vi "Calculate_dx_dy_alpha.vi"(6 "c_y":dbl, 7 "c_x":dbl, 8 "Corresponding Point #2":i32, 9 "Corresponding Point #1":i32, 10 "Original Plots":T1(array[cluster]), 11 "Captured Plots":T1(array[cluster])) -> (1 "alpha":dbl, 2 "dy":dbl, 3 "dx":dbl)   [LabVIEW 2012]
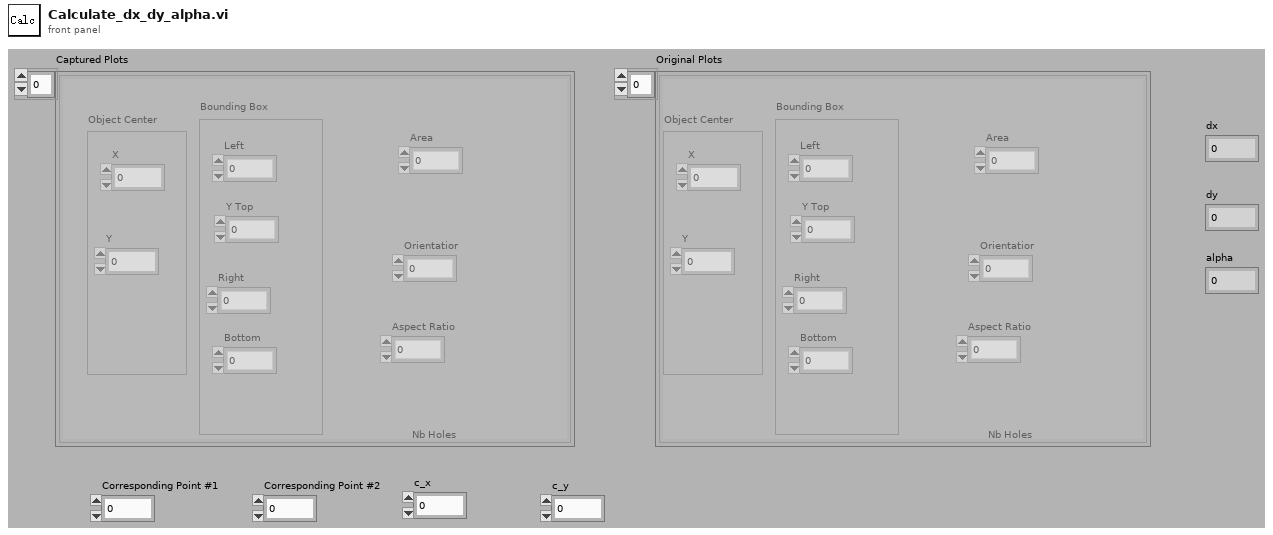
[diagram p1: front panel]
types:
  T1 = cluster{"Object Center":cluster{"X":dbl, "Y":dbl}, "Bounding Box":cluster{"Left":dbl, "Right":dbl, "Bottom":dbl, "Y Top":dbl}, "Area":dbl, "Orientatior":dbl, "Aspect Ratio":dbl, "Nb Holes":dbl}[]
  T2 = cluster{"Object Center":cluster{"X":dbl, "Y":dbl}, "Bounding Box":cluster{"Left":dbl, "Right":dbl, "Bottom":dbl, "Y Top":dbl}, "Area":dbl, "Orientatior":dbl, "Aspect Ratio":dbl, "Nb Holes":dbl}
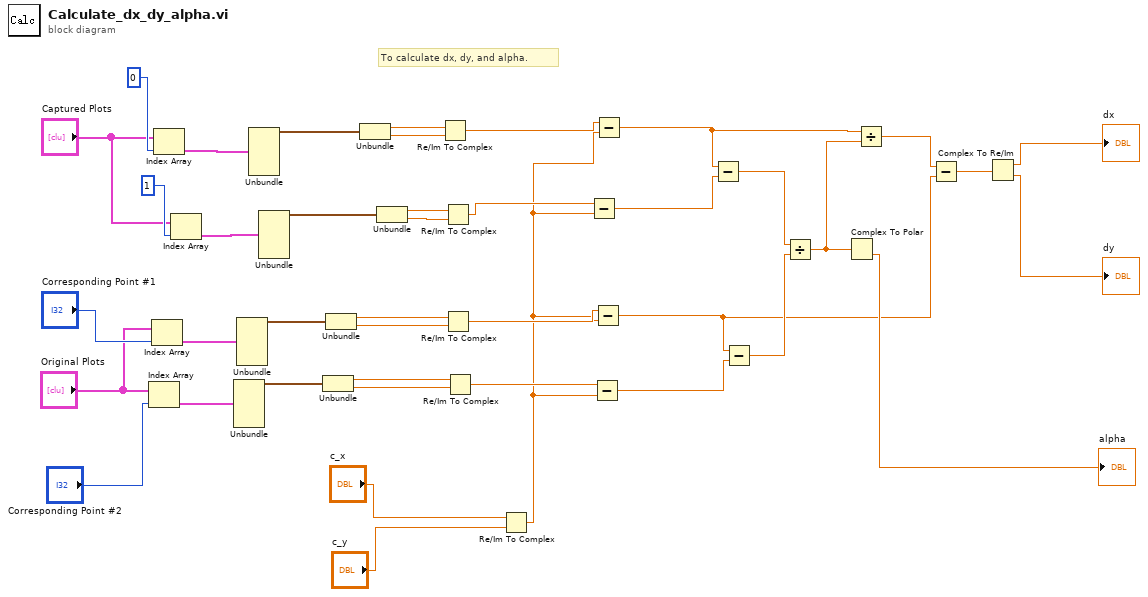
[diagram p0: block diagram]
diagram:
  # "To calculate dx, dy, and alpha."
  n1 = Index Array(array="Original Plots", index="Corresponding Point #2") -> (element=w37:T2)
  n2 = Index Array(array="Original Plots", index="Corresponding Point #1") -> (element=w35:T2)
  n3 = Index Array(array="Captured Plots", index=0) -> (element=w40:T2)
  n4 = Index Array(array="Captured Plots", index=1) -> (element=w31:T2)
  n5 = Unbundle(w37) -> ("Object Center"=w38:cluster{"X":dbl, "Y":dbl})  [unwired: 5 out]
  n6 = Unbundle(w35) -> ("Object Center"=w36:cluster{"X":dbl, "Y":dbl})  [unwired: 5 out]
  n7 = Unbundle(w40) -> ("Object Center"=w39:cluster{"X":dbl, "Y":dbl})  [unwired: 5 out]
  n8 = Unbundle(w31) -> ("Object Center"=w30:cluster{"X":dbl, "Y":dbl})  [unwired: 5 out]
  n9 = Unbundle(w38) -> ("X"=w19:dbl, "Y"=w18:dbl)
  n10 = Unbundle(w36) -> ("X"=w21:dbl, "Y"=w20:dbl)
  n11 = Unbundle(w39) -> ("X"=w25:dbl, "Y"=w24:dbl)
  n12 = Unbundle(w30) -> ("X"=w23:dbl, "Y"=w22:dbl)
  n13 = Re/Im To Complex(1:w24, 2:w25) -> (0:w17:cdb)
  n14 = Re/Im To Complex(1:w22, 2:w23) -> (0:w16:cdb)
  n15 = Re/Im To Complex(1:w20, 2:w21) -> (0:w15:cdb)
  n16 = Re/Im To Complex(1:w18, 2:w19) -> (0:w14:cdb)
  n17 = Re/Im To Complex(1:"c_y", 2:"c_x") -> (0:w13:cdb)
  n18 = Subtract(x=w16, y=w13) -> (x-y=w12:cdb)
  n19 = Subtract(x=w14, y=w13) -> (x-y=w11:cdb)
  n20 = Subtract(x=w15, y=w13) -> (x-y=w4:cdb)
  n21 = Subtract(x=w17, y=w13) -> (x-y=w7:cdb)
  n22 = Subtract(x=w7, y=w12) -> (x-y=w10:cdb)
  n23 = Subtract(x=w4, y=w11) -> (x-y=w9:cdb)
  n24 = Divide(x=w10, y=w9) -> (x/y=w6:cdb)
  n25 = Complex To Polar(r * e^(i*theta)=w6) -> (theta=→"alpha":dbl)  [unwired: 1 out]
  n26 = Divide(x=w7, y=w6) -> (x/y=w5:cdb)
  n27 = Subtract(x=w5, y=w4) -> (x-y=w3:cdb)
  n28 = Complex To Re/Im(x + iy=w3) -> (x=→"dx":dbl, y=→"dy":dbl)
